vi "Pneumatic Command Get Periodic.vi"(11 "Cluster":T1) -> (2 "Status":T2, 3 "Cluster Out":T1)   [LabVIEW 2015]
uses:
  Pneumatics Notifier.ctl
  Pneumatics Command.ctl
  Pneumatics Status.ctl
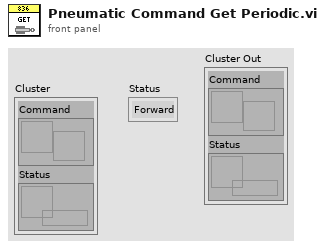
[diagram p1: front panel]
types:
  T1 = typedef "Pneumatics Notifier.ctl" = cluster{"Command":refnum<notifier>, "Status":refnum<queue>}
  T2 = typedef "Pneumatics Status.ctl" = enum16{"Forward", "Reverse", "Moving"}
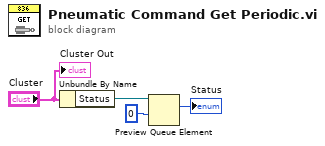
[diagram p0: block diagram]
diagram:
  n1 = Unbundle By Name("Cluster") -> ("Status"=w3:refnum<queue>)
  n2 = Preview Queue Element(queue=w3, timeout in ms (-1)=0) -> (element=→"Status":T2)  [unwired: 1 in, 3 out]
  "Cluster Out" <- "Cluster"
